vi "test Merge Import Status Channels.vi"(8 "error in (no error)":errorcluster, 11 "TestCase in":refnum<class "Routing and Faulting Import Unit Tests.lvclass">) -> (0 "error out":errorcluster, 3 "TestCase out":refnum<class "Routing and Faulting Import Unit Tests.lvclass">)   [LabVIEW 2020, in "Routing and Faulting Import Unit Tests.lvclass"]
uses:
  Routing and Faulting Import Unit Tests.lvclass
  <vilib>/NI VeriStand/Custom Device API/Custom Device Channel.ctl
  <vilib>/NI VeriStand/Custom Device API/Custom Device Channel Type.ctl
  Routing and Faulting Import Unit Tests.lvclass/Routing and Faulting Import Unit Tests.ctl
  <userlib>/_OpenG.lib/file/file.llb/Append Path to Root if Relative - Scalar__ogtk.vi
  <vilib>/addons/_JKI Toolkits/VI Tester/TestCase.llb/TestCase.lvclass
  <vilib>/NI VeriStand/Custom Device Tools/Custom Device Utility Library/Custom Device Utility Library.lvlib
  <vilib>/NI VeriStand/Custom Device API/Custom Device API.lvlib
  niveristand-custom-device-testing-tools/VeriStandTestUtilities/VeriStandTestUtilities.lvlib
  Scripting/Routing and Faulting Scripting.lvlib
  C:/Program Files (x86)/National Instruments/LabVIEW 2020/vi.lib/addons/_JKI Toolkits/VI Tester/TestCase.llb/TestCase.lvclass
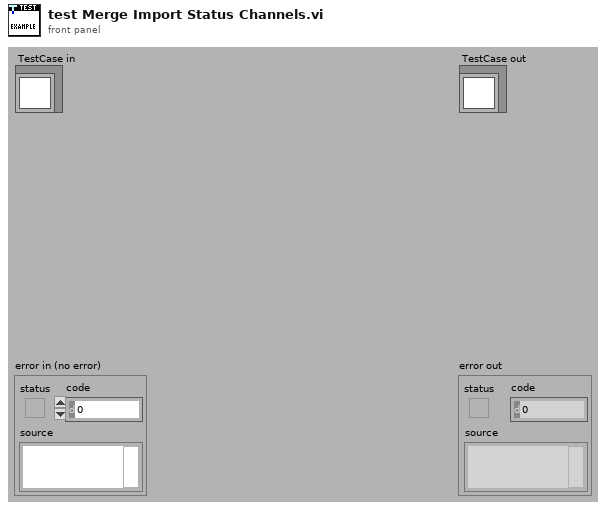
[diagram p1: front panel]
types:
  T1 = typedef "Custom Device API.lvlib/Custom Device Channel.ctl" = cluster{"Type":T2, "Units":string, "Default Value":dbl, "Faultable":bool, "Scalable":bool}
  T2 = typedef "Custom Device API.lvlib/Custom Device Channel Type.ctl" = enum16{"Input", "Output"}
  T3 = typedef "Custom Device API.lvlib/Custom Device Item Ref.ctl" = u64
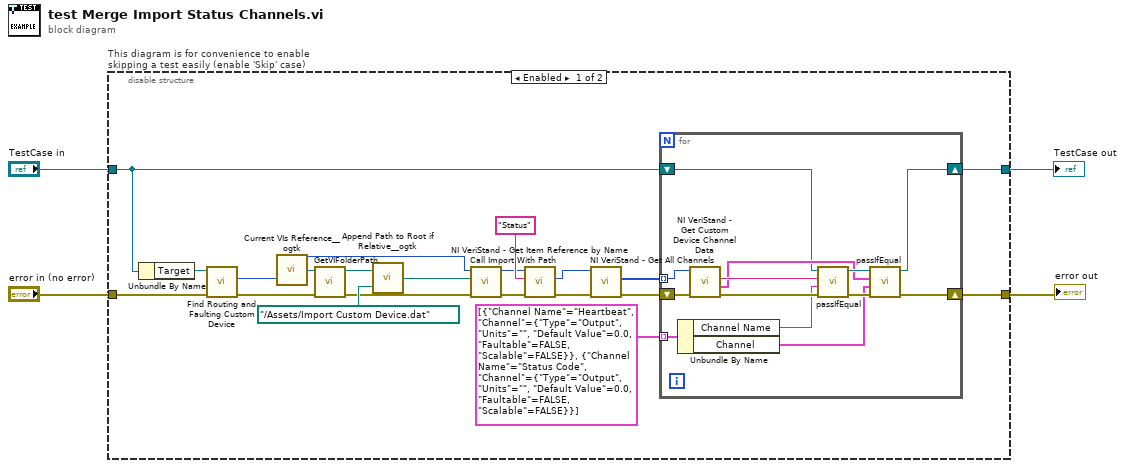
[diagram p0: block diagram]
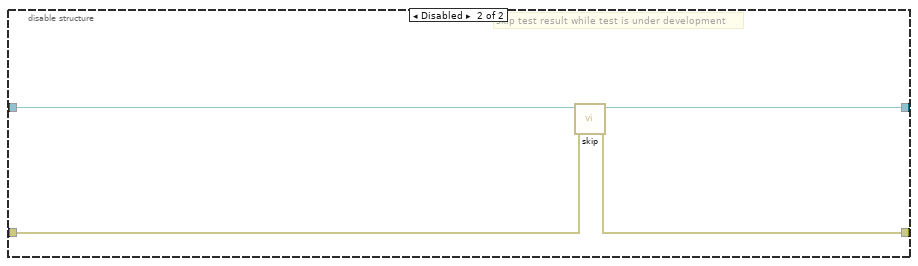
[diagram p2: hidden frame]
diagram:
  n1 = disable-structure "This diagram is for convenience to enable skipping a test easily (enable 'Skip' case)" shown="Enabled" {
    disable-tunnel: "TestCase in" -> [w10 w41]
    disable-tunnel: [w16 w39] -> w1
    disable-tunnel: [w18 w40] -> w3
    disable-tunnel: "error in (no error)" -> [w9 w38]
    frame Enabled {
      n2 = Unbundle By Name(w10) -> ("Target"=w11:refnum<k24>)
      n3 = call "Find Routing and Faulting Custom Device.vi"("error in"=w9, "target in"=w11) -> ("error out"=w12:errorcluster, "routing and faulting custom device"=w6:T3)  [unwired: 7 in, 1 out]
      n4 = call <userlib>:"Current VIs Reference__ogtk.vi"() -> ("Current VI's reference"=w15:refnum<vi>)  [unwired: 5 in]
      n5 = call "GetVIFolderPath.vi"("error in (no error)"=w12, "VI Reference in"=w15) -> ("error out"=w8:errorcluster, "VI Folder Path out"=w14:path)  [unwired: 8 in]
      n6 = call-poly <userlib>:"Append Path to Root if Relative__ogtk.vi"("Absolute or Relative Path"=path "../Assets/Import Custom Device.dat", "Root Path"=w14) -> ("Absolute or Appended Path"=w7:path)
      n7 = call "Call Import With Path.vi"("error in (no error)"=w8, "Path"=w7, "Routing and Faulting Custom Device Ref in"=w6) -> ("error out"=w24:errorcluster, "Routing and Faulting Custom Device Ref out"=w5:T3)  [unwired: 7 in]
      n8 = call <vilib>:"NI VeriStand - Get Item Reference by Name.vi"("error in (no error)"=w24, "Item Name"="Status", "Parent Ref in"=w5) -> ("error out"=w22:errorcluster, "Item Ref"=w21:T3)  [unwired: 5 in, 2 out]
      n9 = call <vilib>:"NI VeriStand - Get All Channels.vi"("error in"=w22, "Section Ref in"=w21) -> ("error out"=w20:errorcluster, "Channel Refs"=w19:T3[])  [unwired: 6 in, 2 out]
      n10 = for {
        shift-right: [w27] -> w18
        shift-left: w20 -> [w37]
        tunnel: w19 -> [w36] mode=indexing
        tunnel: cluster{"Channel Name":string, "Channel":T1}[] [{"Channel Name"="Heartbeat", "Channel"={"Type"=enum."Output", "Units"="", "Default Value"=0.0, "Faultable"=FALSE, "Scalable"=FALSE}}, {"Channel Name"="Status Code", "Channel"={"Type"=enum."Output", "Units"="", "Default Value"=0.0, "Faultable"=FALSE, "Scalable"=FALSE}}] -> [w35] mode=indexing
        shift-right: [w25] -> w16
        shift-left: w10 -> [w26]
        n11 = Unbundle By Name(w35) -> ("Channel Name"=w30:string, "Channel"=w28:T1)
        n12 = call <vilib>:"NI VeriStand - Get Custom Device Channel Data.vi"("error in (no error)"=w37, "Channel Ref in"=w36) -> ("error out"=w34:errorcluster, "Channel"=w29:T1, "Channel Name"=w31:string)  [unwired: 4 in, 3 out]
        n13 = call-dynamic "passIfEqual.vi"("error in (no error)"=w34, "y"=w30, "x"=w31, "TestCase in"=w26) -> ("error out"=w33:errorcluster, "TestCase out"=w32:refnum<class "Routing and Faulting Import Unit Tests.lvclass">)  [unwired: 6 in]
        n14 = call-dynamic "passIfEqual.vi"("error in (no error)"=w33, "y"=w28, "x"=w29, "TestCase in"=w32) -> ("error out"=w27:errorcluster, "TestCase out"=w25:refnum<class "Routing and Faulting Import Unit Tests.lvclass">)  [unwired: 6 in]
      }
    }
    frame Disabled {
      # "skip test result while test is under development"
      n15 = call <vilib>:"skip.vi"("error in (no error)"=w38, "TestCase in"=w41) -> ("error out"=w40:errorcluster, "TestCase out"=w39:refnum<class "Routing and Faulting Import Unit Tests.lvclass">)  [unwired: 8 in]
    }
  }
  "error out" <- w3
  "TestCase out" <- w1
